vi "updateRange.vi"(8 "error in (no error)":errorcluster, 10 "Input Range":dbl=10.0 format="%#_10g", 11 "ElectrometerController in":refnum<class "ElectrometerController.lvclass">) -> (0 "error out":errorcluster, 3 "ElectrometerController out":refnum<class "ElectrometerController.lvclass">)   [LabVIEW 2016, in "ElectrometerController.lvclass"]
uses:
  ElectrometerController.lvclass
  Electrometer/Electrometer.lvclass
  ElectrometerConfiguration/ElectrometerInternalConfiguration.lvclass
  Electrometer/State/ElectrometerState.lvclass
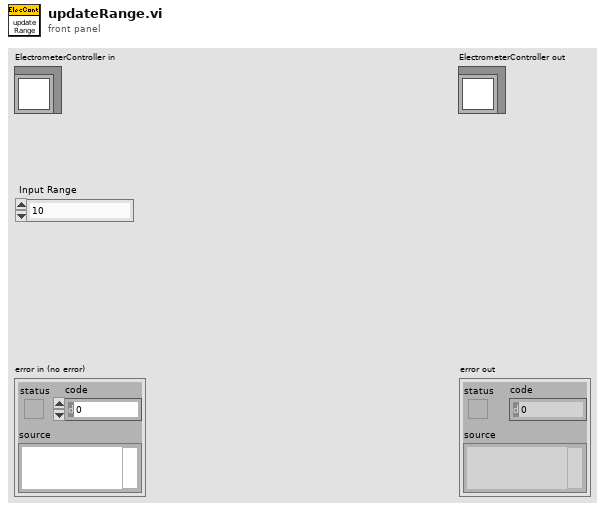
[diagram p1: front panel]
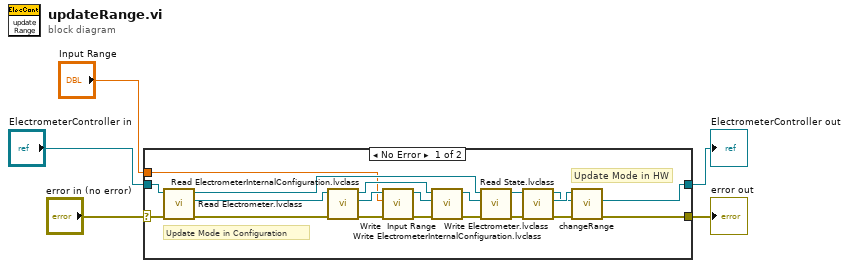
[diagram p0: block diagram]
diagram:
  n1 = case shown="No Error" "error in (no error)" {
    selector: "error in (no error)" -> [w16 w27]
    tunnel: [w7 w27] -> w4
    tunnel: [w6 w26] -> w2
    tunnel: "ElectrometerController in" -> [w17 w26]
    tunnel: "Input Range" -> [w11 _]
    frame No Error {
      # "Update Mode in HW"
      # "Update Mode in Configuration"
      n2 = call-dynamic "Read Electrometer.lvclass.vi"("error in (no error)"=w16, "ElectrometerController in"=w17) -> ("error out"=w18:errorcluster, "Electrometer.lvclass"=w23:refnum<class "Electrometer.lvclass">, "ElectrometerController out"=w22:refnum<class "ElectrometerController.lvclass">)  [unwired: 7 in]
      n3 = call-dynamic "Read ElectrometerInternalConfiguration.lvclass.vi"("error in (no error)"=w18, "Electrometer in"=w23) -> ("error out"=w15:errorcluster, "ElectrometerInternalConfiguration.lvclass"=w12:refnum<class "ElectrometerInternalConfiguration.lvclass">, "Electrometer out"=w25:refnum<class "Electrometer.lvclass">)  [unwired: 7 in]
      n4 = call-dynamic "Write  Input Range .vi"("error in (no error)"=w15, "Input Range"=w11, "ElectrometerInternalConfiguration in"=w12) -> ("error out"=w14:errorcluster, "ElectrometerInternalConfiguration out"=w13:refnum<class "ElectrometerInternalConfiguration.lvclass">)  [unwired: 7 in]
      n5 = call-dynamic "Write ElectrometerInternalConfiguration.lvclass.vi"("error in (no error)"=w14, "ElectrometerInternalConfiguration.lvclass"=w13, "Electrometer in"=w25) -> ("error out"=w21:errorcluster, "Electrometer out"=w24:refnum<class "Electrometer.lvclass">)  [unwired: 7 in]
      n6 = call-dynamic "Write Electrometer.lvclass.vi"("error in (no error)"=w21, "Electrometer.lvclass"=w24, "ElectrometerController in"=w22) -> ("error out"=w20:errorcluster, "ElectrometerController out"=w19:refnum<class "ElectrometerController.lvclass">)  [unwired: 7 in]
      n7 = call-dynamic "Read State.lvclass.vi"("error in (no error)"=w20, "ElectrometerController in"=w19) -> ("error out"=w8:errorcluster, "ElectrometerState"=w10:refnum<class "ElectrometerState.lvclass">, "ElectrometerController out"=w9:refnum<class "ElectrometerController.lvclass">)  [unwired: 7 in]
      n8 = call-dynamic "changeRange.vi"("error in (no error)"=w8, "ElectrometerController in"=w9, "ElectrometerState in"=w10) -> ("error out"=w7:errorcluster, "ElectrometerController out"=w6:refnum<class "ElectrometerController.lvclass">)  [unwired: 6 in, 1 out]
    }
    frame Error {
    }
  }
  "error out" <- w4
  "ElectrometerController out" <- w2
